vi "Execute Build.vi"(0 "CLI in":refnum<class "CLI.lvclass">, 5 "All Build Specs":string[](array[string]), 7 "Proj Path":path, 11 "error in (no error)":errorcluster, 12 "Targets":string[](array[string])) -> (4 "CLI out":refnum<class "CLI.lvclass">, 6 "Created Files":path[](array[path]), 15 "error out":errorcluster)   [LabVIEW 2023]
doc: "Execute Build.vi\n----------------------------------------------\nThis SubVI executes the actual build\n\nInputs:\n---------------------\n- All Build Specs : 1DArrayOfString; \n- Proj Path : Path; \n- CLI in : LabVIEW Class Instance; \n- error in (no error) : Cluster; \n- Specs to be built : 1DArrayOfI32; \n\nOutputs:\n---------------------\n- error out : Cluster; \n- CLI out : LabVIEW Class Instance; \n- Created Files : 1DArrayOfPath; \n\n----------------------------------------------\n6/1/2021 nina\nZühlke Engineering AG\nCH-8952 Schlieren\nwww.zuehlke.com"
uses:
  <vilib>/Wiresmith Technology/G CLI/CLI Class/CLI.lvclass
  <vilib>/AppBuilder/AB_API_Simple/Build (path).vi
  <vilib>/AppBuilder/AB_API_Simple/NI_App_Builder_API.lvlib
panel:
  # "Connector Pane"
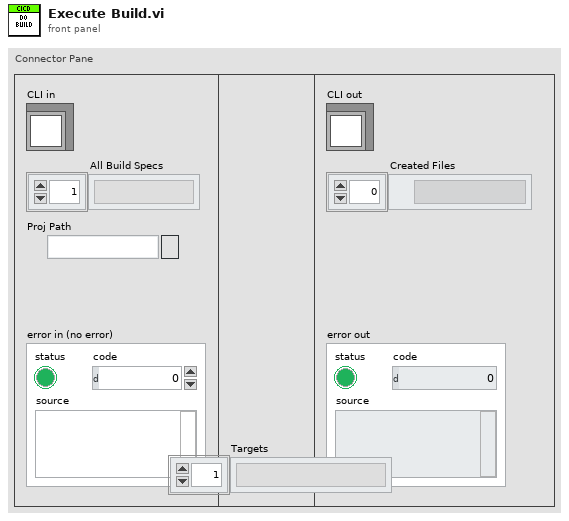
[diagram p1: front panel]
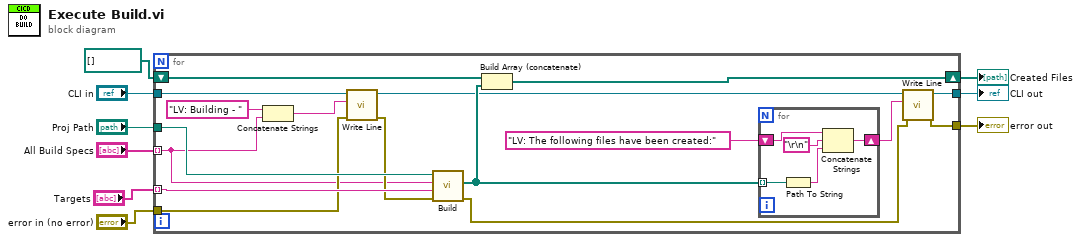
[diagram p0: block diagram]
diagram:
  n1 = for {
    tunnel: "Proj Path" -> [w26]
    tunnel: "CLI in" -> [w15]
    tunnel: [w25] -> w8
    tunnel: "error in (no error)" -> [w14]
    tunnel: [w21] -> w9
    tunnel: "All Build Specs" -> [w10] mode=indexing
    shift-right: [w19] -> w7
    shift-left: path[] [] -> [w18]
    tunnel: "Targets" -> [w17] mode=indexing
    n2 = Concatenate Strings("LV: Building - " ("Text to Write"), w10) -> (w12:string)
    n3 = call <vilib>:"Write Line.vi"("error in (no error)"=w14, "Text to Write"=w12, "CLI in"=w15) -> ("error out"=w13:errorcluster, "CLI out"=w16:refnum<class "CLI.lvclass">)  [unwired: 7 in]
    n4 = call-poly <vilib>:"Build.vi"("error in (no error)"=w13, "Name of target (My Computer)"=w17, "Name of build specification (if empty: build all)"=w10, "Path to project"=w26) -> ("error out"=w22:errorcluster, "Generated files"=w20:path[])  [unwired: 6 in]
    n5 = Build Array (concatenate)(w18, w20) -> (w19:path[])
    n6 = for {
      tunnel: w20 -> [w29] mode=indexing
      shift-right: [w27] -> w23
      shift-left: "LV: The following files have been created:" ("Text to Write") -> [w31]
      n7 = Path To String(path=w29) -> (string=w28:string)
      n8 = Concatenate Strings(w31, "\r\n", w28) -> (w27:string)
    }
    n9 = call <vilib>:"Write Line.vi"("error in (no error)"=w22, "Text to Write"=w23, "CLI in"=w16) -> ("error out"=w21:errorcluster, "CLI out"=w25:refnum<class "CLI.lvclass">)  [unwired: 7 in]
  }
  "error out" <- w9
  "CLI out" <- w8
  "Created Files" <- w7
